vi "positionChooseMarker.vi"(5 "enemyRobots":refnum<class "Robot.lvclass">[](array[class]), 7 "OffensiveRobots":refnum<class "Robot.lvclass">[](array[class]), 8 "error in (no error)":errorcluster, 10 "dangerEnemies in":T1[](array[typedef]), 11 "MarkerSkill in":refnum<class "MarkerSkill.lvclass">) -> (0 "error out":errorcluster, 2 "dangerEnemies out":T1[](array[typedef]), 3 "MarkerSkill out":refnum<class "MarkerSkill.lvclass">)   [LabVIEW 2020, in "MarkerSkill.lvclass"]
uses:
  MarkerSkill.lvclass
  Robot_class/Robot.lvclass
  C:/RoboIME/SSL_AI/Object_class/Object.lvclass
  dangerEnemy.ctl
  Object_class/Object.lvclass/Object.ctl
  Object_class/Read position(x,y).vi
  Utilities_class/Utilities.lvclass
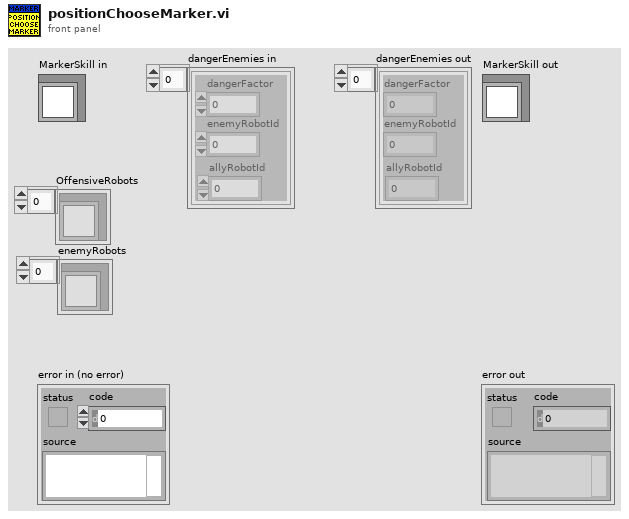
[diagram p1: front panel]
types:
  T1 = typedef "dangerEnemy.ctl" = cluster{"dangerFactor":dbl, "allyRobotId":i32, "enemyRobotId":i32}
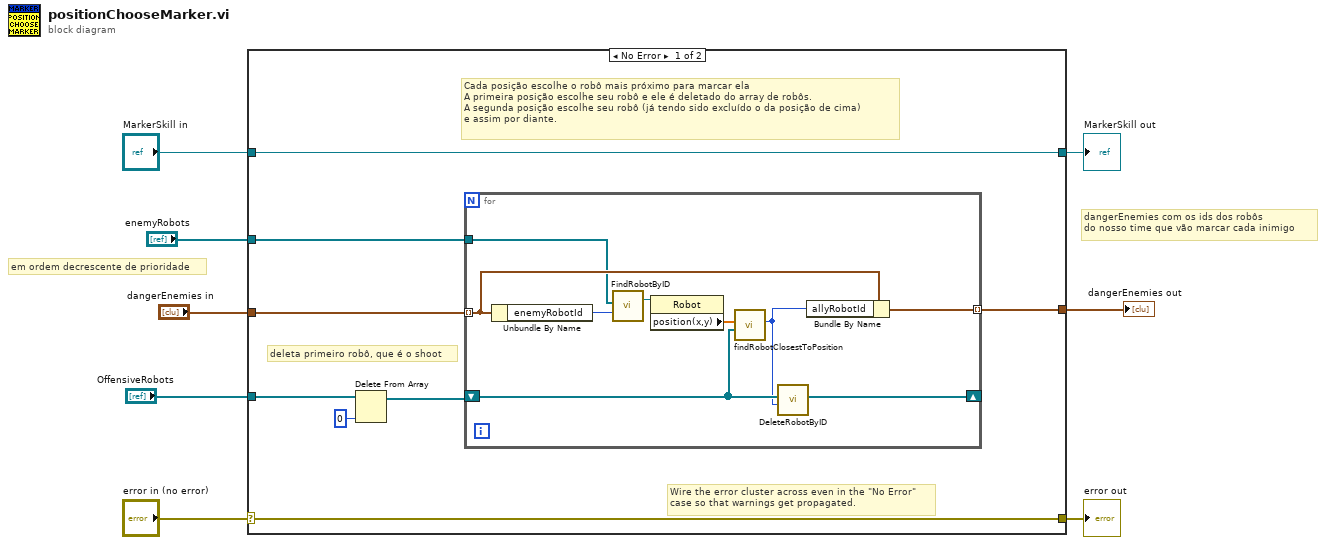
[diagram p0: block diagram]
diagram:
  # "dangerEnemies com os ids dos robôs\ndo nosso time que vão marcar cada inimigo"
  # "em ordem decrescente de prioridade"
  n1 = case shown="No Error" "error in (no error)" {
    selector: "error in (no error)" -> [w15 w27]
    tunnel: [w15 w27] -> w7
    tunnel: [w16 w26] -> w5
    tunnel: "MarkerSkill in" -> [w16 w26]
    tunnel: "OffensiveRobots" -> [w14 _]
    tunnel: "dangerEnemies in" -> [w11 _]
    tunnel: [w10 _] -> w2
    tunnel: "enemyRobots" -> [w9 _]
    frame No Error {
      # "Cada posição escolhe o robô mais próximo para marcar ela\nA primeira posição escolhe seu robô e ele é deletado do array de robôs.\nA segunda posição escolhe seu robô (já tendo sido excluído o da posição de cima)\ne assim por diante."
      # "deleta primeiro robô, que é o shoot"
      # "Wire the error cluster across even in the \"No Error\"\ncase so that warnings get propagated."
      n2 = Delete From Array(array=w14, index=0) -> (array with subset deleted=w13:refnum<class "Robot.lvclass">[])  [unwired: 1 in, 1 out]
      n3 = for {
        tunnel: w11 -> [w22] mode=indexing
        tunnel: [w21] -> w10 mode=indexing
        shift-right: [w18] -> _
        shift-left: w13 -> [w20]
        tunnel: w9 -> [w17]
        n4 = Unbundle By Name(w22) -> ("enemyRobotId"=w25:i32)
        n5 = call "FindRobotByID.vi"("id"=w25, "RobotRef"=w17) -> ("Robot"=w24:refnum<class "Robot.lvclass">)  [unwired: 6 in, 3 out]
        n6 = property class="Robot"(reference=w24) -> ("position(x,y)"=w23:dbl[])  [unwired: 1 in, 2 out]
        n7 = call "findRobotClosestToPosition.vi"("robotsArray"=w20, "position"=w23) -> ("id"=w19:i32)  [unwired: 5 in, 4 out]
        n8 = call "DeleteRobotByID.vi"("id"=w19, "RobotRef"=w20) -> ("RobotRef out"=w18:refnum<class "Robot.lvclass">[])  [unwired: 7 in, 2 out]
        n9 = Bundle By Name(cluster=w22, "allyRobotId"=w19) -> (w21:T1)
      }
    }
    frame Error {
    }
  }
  "error out" <- w7
  "MarkerSkill out" <- w5
  "dangerEnemies out" <- w2
